vi "Read File.vi"(8 "error in (no error)":errorcluster, 10 "Path":path, 11 "Read Config File in":refnum<class "Read Config File.lvclass">) -> (0 "error out":errorcluster, 3 "Read Config File out":refnum<class "Read Config File.lvclass">)   [LabVIEW 2025, in "Config Library.lvlib" / "Read Config File.lvclass"]
uses:
  Read Config File.lvclass
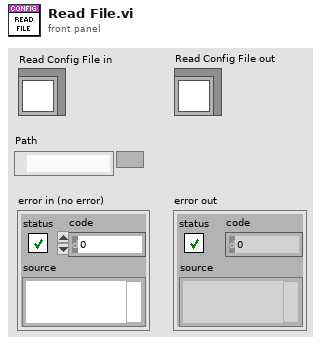
[diagram p1: front panel]
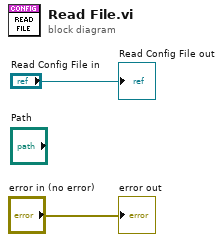
[diagram p0: block diagram]
diagram:
  "error out" <- "error in (no error)"
  "Read Config File out" <- "Read Config File in"
